vi "StreamCtrl.vi"(8 "error in (no error)":errorcluster, 9 "StreamValue":T1, 10 "Enable":bool, 11 "MFActor in":refnum<class "MFActor.lvclass">) -> (0 "error out":errorcluster, 3 "MFActor out":refnum<class "MFActor.lvclass">)   [LabVIEW 2024, in "MFActor.lvlib" / "MFActor.lvclass"]
uses:
  MFActor.lvclass
  MFActor.lvclass/MFActor.ctl
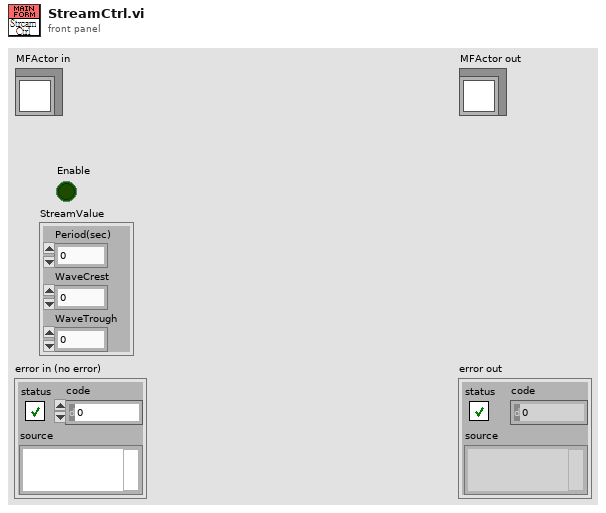
[diagram p1: front panel]
types:
  T1 = cluster{"Period(sec)":dbl, "WaveCrest":dbl, "WaveTrough":dbl}
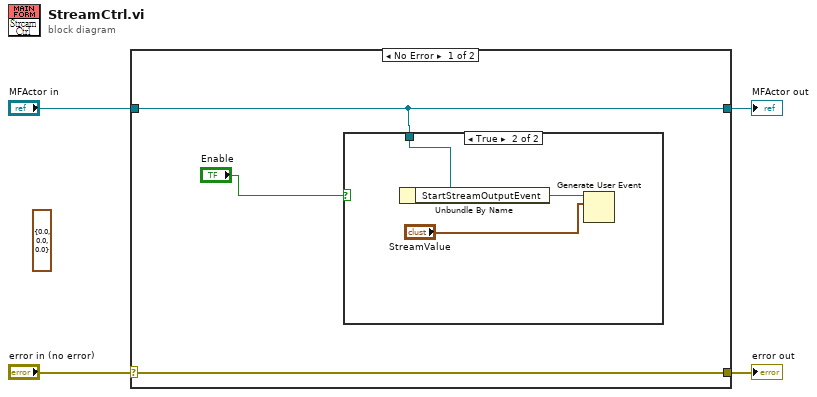
[diagram p0: block diagram]
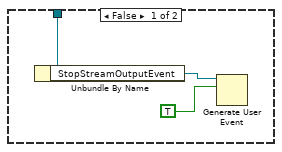
[diagram p2: hidden frame]
diagram:
  (unwired) T1 {"Period(sec)"=0.0, "WaveCrest"=0.0, "WaveTrough"=0.0} ("StreamValue")
  n1 = case shown="No Error" "error in (no error)" {
    selector: "error in (no error)" -> [w7 w15]
    tunnel: [w7 w15] -> w3
    tunnel: [w5 w14] -> w1
    tunnel: "MFActor in" -> [w5 w14]
    frame No Error {
      n2 = case shown="True" "Enable" {
        tunnel: w5 -> [w10 w13]
        frame False {
          n3 = Unbundle By Name(w10) -> ("StopStreamOutputEvent"=w9:refnum<user-event>)
          n4 = Generate User Event(user event=w9, event data cluster=TRUE ("event data")) -> ()  [unwired: 2 in, 2 out]
        }
        frame True {
          n5 = Unbundle By Name(w13) -> ("StartStreamOutputEvent"=w12:refnum<user-event>)
          n6 = Generate User Event(user event=w12, event data cluster="StreamValue") -> ()  [unwired: 2 in, 2 out]
        }
      }
    }
    frame Error {
    }
  }
  "error out" <- w3
  "MFActor out" <- w1
